vi "SR Disable.vi"(8 "error in":errorcluster, 10 "SR":string, 11 "specific class reference":refnum<vi>) -> (0 "error out":errorcluster)   [LabVIEW 2019, in "Inst UI.Krohn-Hite-7008.lvclass"]
uses:
  Inst UI.Krohn-Hite-7008.lvclass
  KH7008/typedefs/shunt--enum.ctl
  KH7008/KH7008.lvlib
panel:
  in  "demo Shunt Resistor":T1=enum."50"
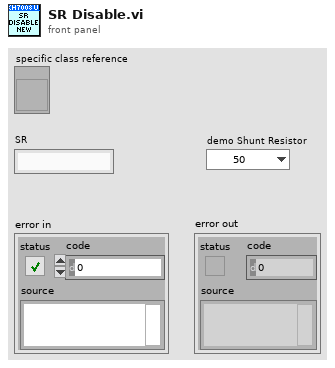
[diagram p1: front panel]
types:
  T1 = typedef "KH7008.lvlib/shunt--enum.ctl" = enum16{"Open", "50", "500", "5k", "50k", "10M"}
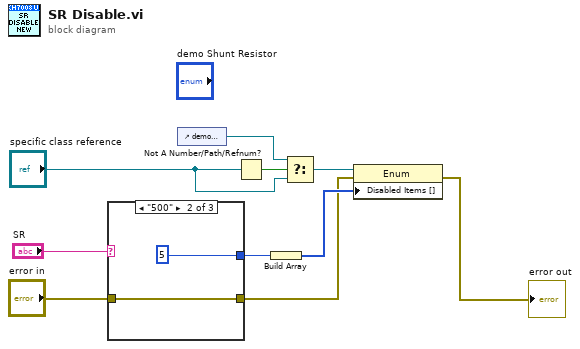
[diagram p0: block diagram]
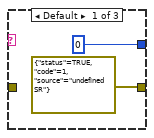
[diagram p2: hidden frame]
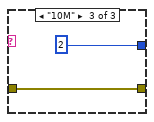
[diagram p3: hidden frame]
diagram:
  n1 = case shown="\"500\"" "SR" {
    tunnel: [0 5 2] -> w10
    tunnel: "error in" -> [_ w13 w15]
    tunnel: [errorcluster {"status"=TRUE, "code"=1, "source"="undefined SR"} ("error in") w13 w15] -> w1
    frame Default {
    }
    frame "500" {
    }
    frame "10M" {
    }
  }
  n2 = control-ref of="demo Shunt Resistor"() -> (w5:refnum<vi>)
  n3 = Not A Number/Path/Refnum?(number/path/refnum="specific class reference") -> (NaN/Path/Refnum?=w8:bool)
  n4 = Build Array(w10) -> (w9:i32[])
  n5 = Select(t=w5, s=w8, f="specific class reference") -> (s? t:f=w7:refnum<vi>)
  n6 = property class="Enum"(reference=w7, error in=w1, "Disabled Items []"=w9) -> (error out=→"error out":errorcluster)  [unwired: 1 out]
